vi "NT IsConnected.vi"() -> (0 "Error":errorcluster={"status"=FALSE, "code"=-1, "source"=""}, 3 "Connected":bool)   [LabVIEW 2025]
doc: "Place this VI in the Dashboard or other client applications. Provide the robot IP address so that it can know where to find the server.\n\nYou normally want the restart option to be true, but if you have your own restart strategy, you can disable it. Tracing is useful when debugging. Similarly, the disconnect timout may need to be raised if setting breakpoints. The user event ref will publish the client activities so that other elements of the dashboard are notified when packets are processed."
uses:
  ntcoreffi.dll
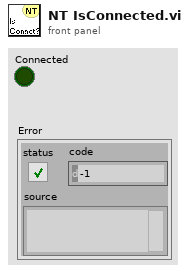
[diagram p1: front panel]
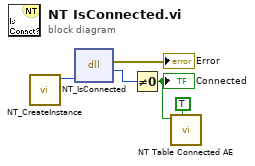
[diagram p0: block diagram]
diagram:
  n1 = call <vilib>:"NT_CreateInstance.vi"() -> ("InstanceHandle"=w4:u64)  [unwired: 10 in, 1 out]
  n2 = dll-call lib="ntcoreffi.*" fn="NT_IsConnected"("inst"=w4) -> (error out=→"Error":errorcluster, "return type"=w3:u32)  [unwired: 4 in, 1 out]
  n3 = Not Equal To 0?(x=w3) -> (x != 0?=w2:bool)
  "Connected" <- w2
  n4 = call "NT Table Connected AE.vi"("Update"=TRUE, "NT Table Connected in"=w2) -> ()  [unwired: 9 in, 1 out]
